vi "Scope_FPGA_Cavities_v00.vi"(0 "Scope IPs":T12, 9 "Scope":T8, 11 "Lock 4":T1, 12 "Cavities Data":u64[](array[numeric])) -> (3 "Scope OP Graph":cluster{dbl[], dbl[]}[](graph), 4 "Scope Cavities ON":bool, 8 "error":dbl[](array[numeric]), 10 "Scope Cavities":T13)   [LabVIEW 2010]
doc: "Creates an oscilliscope graph from the FIFO data, as well as packages data structures for FPGA_Cavities via the reference. (Needs tidying up). Based on a design by Ben Sparkes."
uses:
  Strict Type Defs/Control GUI v01.ctl
  Strict Type Defs/Slider and display.ctl
  Strict Type Defs/I16 white control.ctl
  Strict Type Defs/PII Gains.ctl
  Strict Type Defs/I2 gain slider.ctl
  Strict Type Defs/Thresh slider.ctl
  Strict Type Defs/Lock or Hold.ctl
  Strict Type Defs/Scan Freq Slider.ctl
  Strict Type Defs/DC polarity.ctl
  Strict Type Defs/Gains negative vertical.ctl
  Strict Type Defs/Lock Select 4.ctl
panel:
  in  "OPO A":T2={"Offset Error"=-0.004322033898305084, "Gain Error"=1, "Offset DC"=0.18926553672316412, "Gain DC"=1, "P Gain"=12, "P Bit Shift"=-7, "I Bit Shift"=-7, "I2 Bit Shift"=-27, "I Gain"=19, "I2 Gain"=0, "Lock Threshold"=66, "Lock"=FALSE, "Hold"=FALSE, "Scan Frequency"=19, "Scan Bit Shift"=-4, "DC negative"=FALSE, "Gains -ve "=FALSE} {"Scan Frequency" scale=1.0..30.0; "I2 Gain" scale=0.0..10.0; "I Gain" scale=0.0..50.0; "P Gain" scale=0.0..50.0; "Offset DC" scale=-5.0..0.5 scale format="%#_5f"; "Offset Error" scale=-0.01..0.005 scale format="%#_5f"}
  in  "OPO B":T2={"Offset Error"=-0.011977401129943503, "Gain Error"=4, "Offset DC"=1.29177966101695, "Gain DC"=1, "P Gain"=14, "P Bit Shift"=-8, "I Bit Shift"=-8, "I2 Bit Shift"=-27, "I Gain"=13, "I2 Gain"=0, "Lock Threshold"=67, "Lock"=FALSE, "Hold"=FALSE, "Scan Frequency"=10, "Scan Bit Shift"=-5, "DC negative"=TRUE, "Gains -ve "=FALSE} {"Scan Frequency" scale=1.0..30.0; "I2 Gain" scale=0.0..10.0; "I Gain" scale=0.0..50.0; "P Gain" scale=0.0..50.0; "Offset DC" scale=-5.1..3.0 scale format="%#_5f"; "Offset Error" scale format="%#_5f"}
  in  "MCC":T2={"Offset Error"=-0.006610169491525424, "Gain Error"=1, "Offset DC"=0.028813559322033905, "Gain DC"=1, "P Gain"=14, "P Bit Shift"=-8, "I Bit Shift"=-11, "I2 Bit Shift"=-27, "I Gain"=11, "I2 Gain"=0, "Lock Threshold"=20, "Lock"=FALSE, "Hold"=FALSE, "Scan Frequency"=10, "Scan Bit Shift"=-4, "DC negative"=TRUE, "Gains -ve "=TRUE} {"Scan Frequency" scale=1.0..30.0; "I2 Gain" scale=0.0..10.0; "I Gain" scale=0.0..50.0; "P Gain" scale=0.0..50.0; "Offset DC" scale=-0.1..0.2 scale format="%#_5f"; "Offset Error" scale=-0.02..0.01 scale format="%#_5f"}
  in  "Doubler":T2={"Offset Error"=-0.011581920903954804, "Gain Error"=1, "Offset DC"=-0.023163841807909608, "Gain DC"=1, "P Gain"=10, "P Bit Shift"=-7, "I Bit Shift"=-8, "I2 Bit Shift"=-27, "I Gain"=21, "I2 Gain"=0, "Lock Threshold"=12, "Lock"=FALSE, "Hold"=FALSE, "Scan Frequency"=8, "Scan Bit Shift"=-5, "DC negative"=FALSE, "Gains -ve "=FALSE} {"Scan Frequency" scale=1.0..30.0; "I2 Gain" scale=0.0..10.0; "I Gain" scale=0.0..50.0; "P Gain" scale=0.0..50.0; "Offset DC" scale=-0.1..0.1 scale format="%#_5f"; "Offset Error" scale=-0.05..0.05 scale format="%#_5f"}
  out "Scope OPs (for saving)":cluster{dbl[], i16[], i16[], i16[], i16[]}
  in  "Scope":T13={"Trigger Direction"=enum."minus-plus", "Delay"=0, "Aquisition Rate (Ticks)"=20, "Offset"=0, "Channel"=0, "Channel Selector"={"Channel 1"=0, "Channel 2"=0, "Channel 3"=0, "Channel 4"=0}}
  # "PII Gains"
  # "Lock"
  # "Error Signal"
  # "Monitor"
  # "Scan"
  # "DC positive"
  # "PII Gains"
  # "Lock"
  # "Error Signal"
  # "Monitor"
  # "Scan"
  # "DC positive"
  # "PII Gains"
  # "Lock"
  # "Error Signal"
  # "Monitor"
  # "Scan"
  # "DC positive"
  # "PII Gains"
  # "Lock"
  # "Error Signal"
  # "Monitor"
  # "Scan"
  # "DC positive"
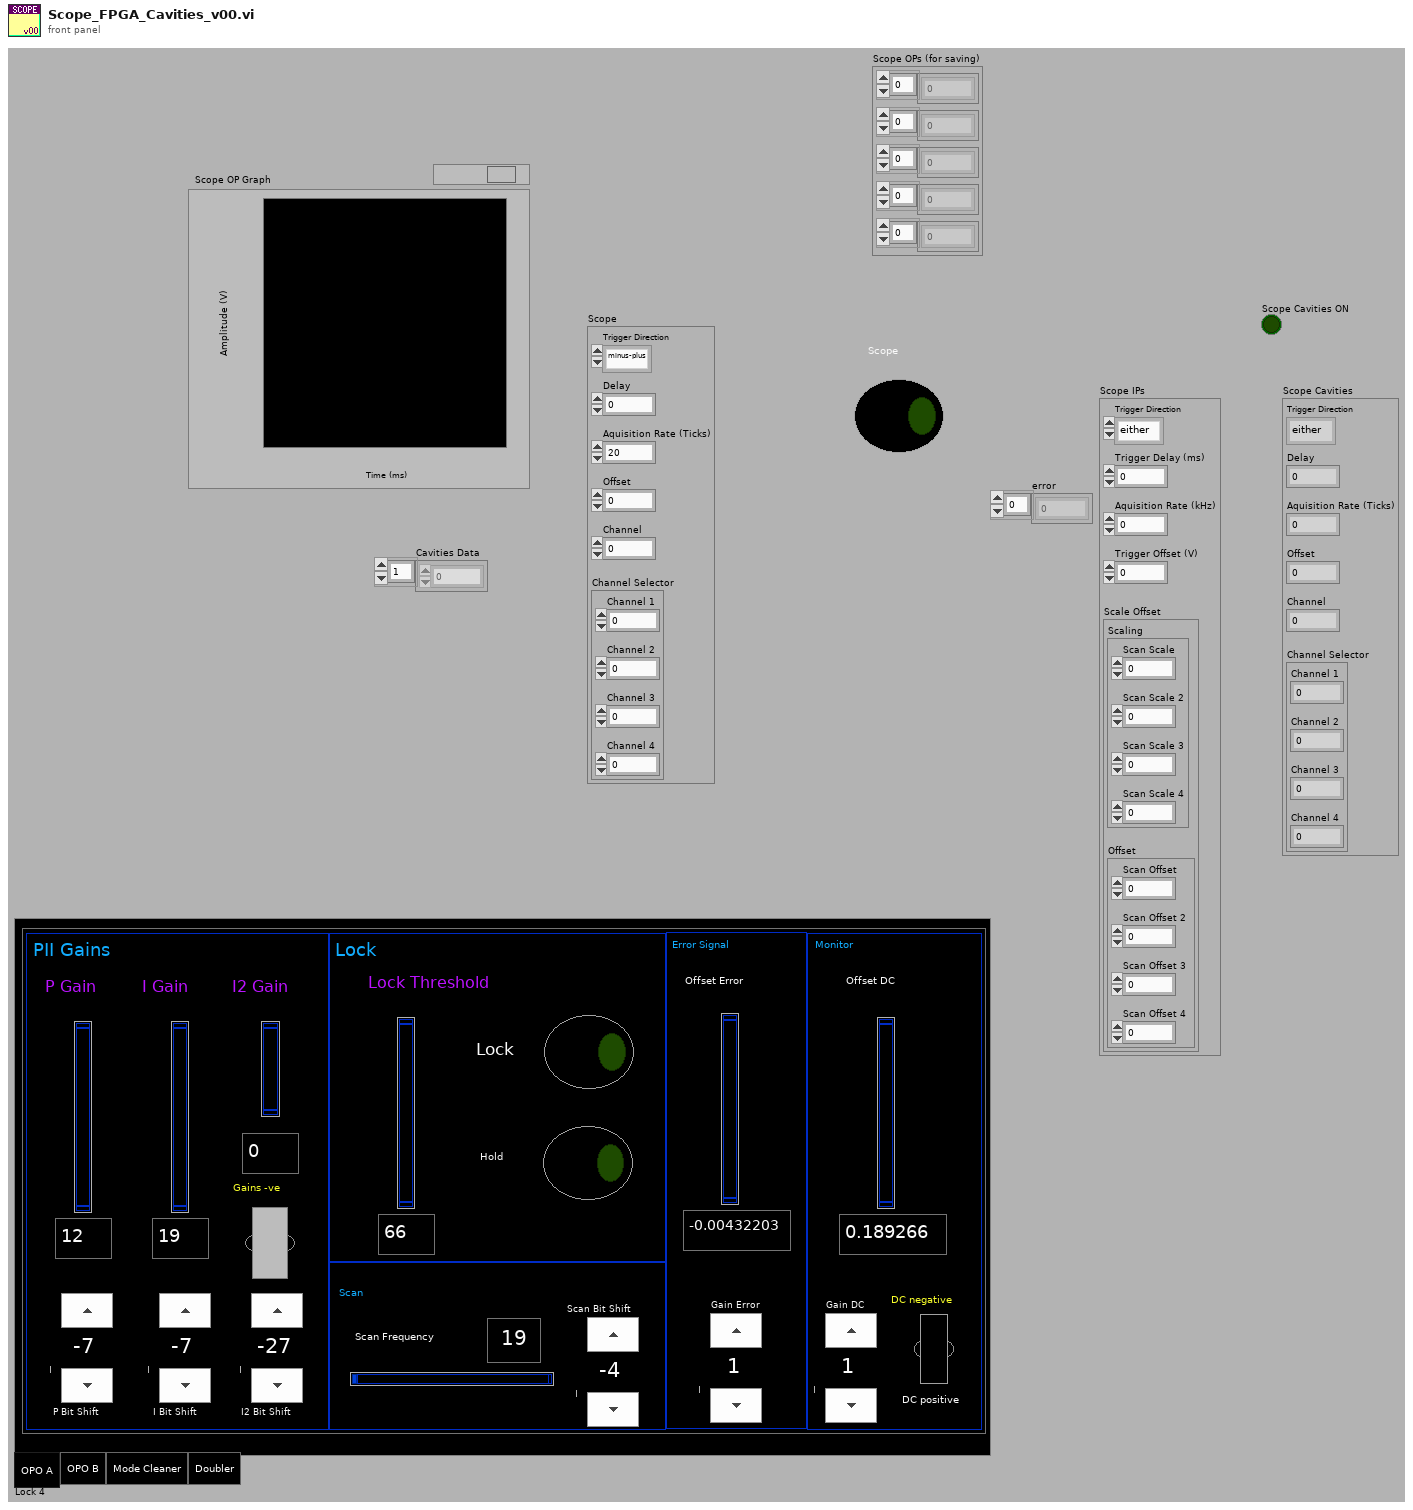
[diagram p1: front panel]
types:
  T1 = typedef "Lock Select 4.ctl" = enum32{"OPO A", "OPO B", "Mode Cleaner", "Doubler"}
  T2 = typedef "Control GUI v01.ctl" = cluster{"Offset Error":T3, "Gain Error":T4, "Offset DC":T3, "Gain DC":T4, "P Gain":T5, "P Bit Shift":T4, "I Bit Shift":T4, "I2 Bit Shift":T4, "I Gain":T5, "I2 Gain":T6, "Lock Threshold":T7, "Lock":T8, "Hold":T8, "Scan Frequency":T9, "Scan Bit Shift":T4, "DC negative":T10, "Gains -ve ":T11}
  T3 = typedef "Slider and display.ctl" = dbl
  T4 = typedef "I16 white control.ctl" = i16
  T5 = typedef "PII Gains.ctl" = i32
  T6 = typedef "I2 gain slider.ctl" = i32
  T7 = typedef "Thresh slider.ctl" = i16
  T8 = typedef "Lock or Hold.ctl" = bool
  T9 = typedef "Scan Freq Slider.ctl" = u16
  T10 = typedef "DC polarity.ctl" = bool
  T11 = typedef "Gains negative vertical.ctl" = bool
  T12 = cluster{"Trigger Direction":enum8{"either", "minus-plus", "plus-minus"}, "Trigger Delay (ms)":dbl, "Aquisition Rate (kHz)":dbl, "Trigger Offset (V)":dbl, "Scale Offset":cluster{"Scaling":cluster{"Scan Scale":i16, "Scan Scale 2":i16, "Scan Scale 3":i16, "Scan Scale 4":i16}, "Offset":cluster{"Scan Offset":i16, "Scan Offset 2":i16, "Scan Offset 3":i16, "Scan Offset 4":i16}}}
  T13 = cluster{"Trigger Direction":enum8{"either", "minus-plus", "plus-minus"}, "Delay":u32, "Aquisition Rate (Ticks)":u32, "Offset":i16, "Channel":i32, "Channel Selector":cluster{"Channel 1":i32, "Channel 2":i32, "Channel 3":i32, "Channel 4":i32}}
  T14 = cluster{"Channel 1":i32, "Channel 2":i32, "Channel 3":i32, "Channel 4":i32}
  T15 = cluster{"Scan Scale":i16, "Scan Scale 2":i16, "Scan Scale 3":i16, "Scan Scale 4":i16}
  T16 = cluster{"Scan Offset":i16, "Scan Offset 2":i16, "Scan Offset 3":i16, "Scan Offset 4":i16}
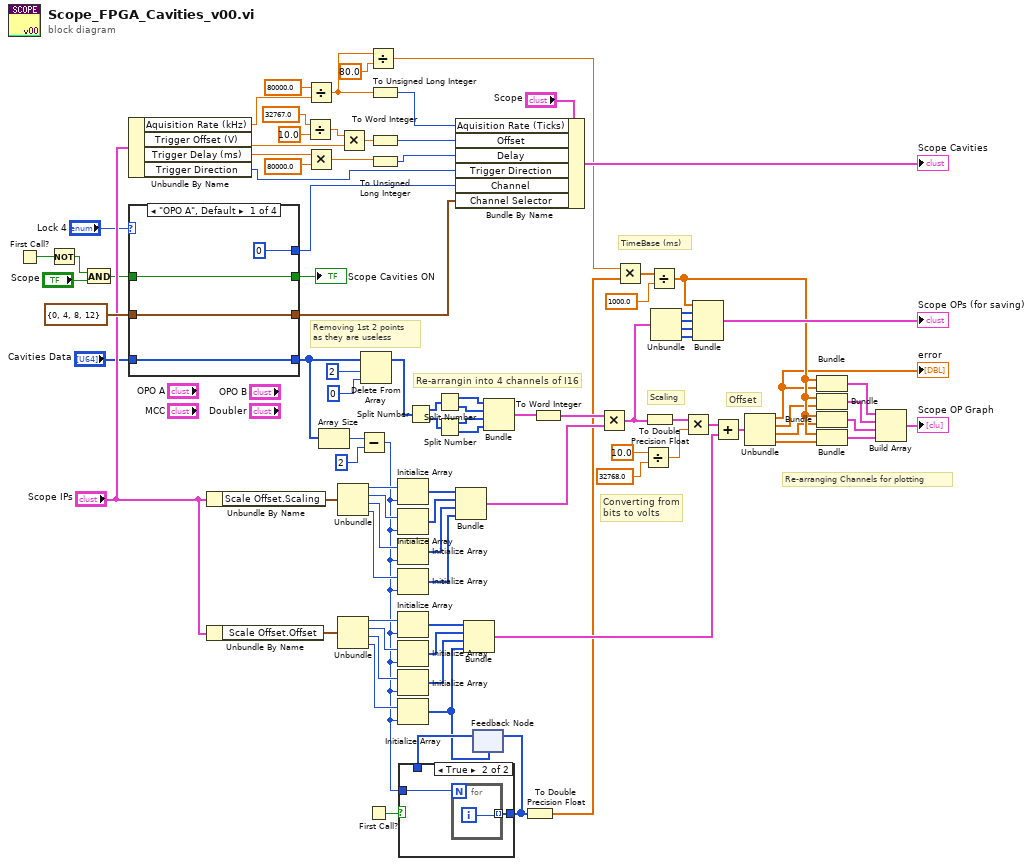
[diagram p0: block diagram]
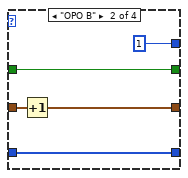
[diagram p3: hidden frame]
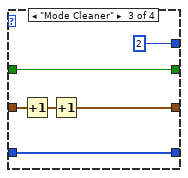
[diagram p4: hidden frame]
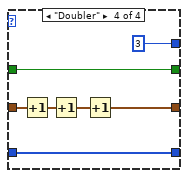
[diagram p5: hidden frame]
diagram:
  # "TimeBase (ms)"
  # "Re-arranging Channels for plotting"
  # "Re-arrangin into 4 channels of I16"
  # "Converting from\nbits to volts"
  # "Offset"
  # "Scaling"
  # "Removing 1st 2 points\nas they are useless"
  n1 = First Call?() -> (First Call?: T/F=w9:bool)
  n2 = Not(x=w9) -> (.not. x?=w4:bool)
  n3 = And(x=w4, y="Scope") -> (x .and. y?=w7:T8)
  n4 = Unbundle By Name("Scope IPs") -> ("Aquisition Rate (kHz)"=w92:dbl, "Trigger Offset (V)"=w87:dbl, "Trigger Delay (ms)"=w85:dbl, "Trigger Direction"=w10:enum8{"either", "minus-plus", "plus-minus"})
  n5 = case shown="\"OPO A\", Default" "Lock 4" {
    tunnel: T14 {"Channel 1"=0, "Channel 2"=4, "Channel 3"=8, "Channel 4"=12} ("Channel Selector") -> [w97 w100 w106 w113]
    tunnel: [w97 w99 w104 w110] -> w83
    tunnel: [0 1 2 3] -> w82
    tunnel: [w96 w102 w108 w115] -> w16
    tunnel: "Cavities Data" -> [w96 w102 w108 w115]
    tunnel: [w94 w98 w103 w109] -> w8
    tunnel: w7 -> [w94 w98 w103 w109]
    frame "OPO A", Default {
    }
    frame "OPO B" {
      n6 = Increment(x=w100) -> (x+1=w99:T14)
    }
    frame "Mode Cleaner" {
      n7 = Increment(x=w106) -> (x+1=w105:T14)
      n8 = Increment(x=w105) -> (x+1=w104:T14)
    }
    frame "Doubler" {
      n9 = Increment(x=w113) -> (x+1=w112:T14)
      n10 = Increment(x=w112) -> (x+1=w111:T14)
      n11 = Increment(x=w111) -> (x+1=w110:T14)
    }
  }
  "Scope Cavities ON" <- w8
  n12 = Unbundle By Name("Scope IPs") -> ("Scale Offset.Scaling"=w47:T15)
  n13 = Unbundle By Name("Scope IPs") -> ("Scale Offset.Offset"=w31:T16)
  n14 = Divide(x=32767.0, y=10.0) -> (x/y=w90:dbl)
  n15 = Divide(x=80000.0, y=w92) -> (x/y=w80:dbl)
  n16 = Multiply(x=w85, y=80000.0) -> (x*y=w86:dbl)
  n17 = Array Size(array=w16) -> (size(s)=w76:i32)
  n18 = Unbundle(w47) -> ("Scan Scale"=w44:i16, "Scan Scale 2"=w43:i16, "Scan Scale 3"=w45:i16, "Scan Scale 4"=w46:i16)
  n19 = Unbundle(w31) -> ("Scan Offset"=w30:i16, "Scan Offset 2"=w34:i16, "Scan Offset 3"=w33:i16, "Scan Offset 4"=w32:i16)
  n20 = Multiply(x=w90, y=w87) -> (x*y=w91:dbl)
  n21 = Subtract(x=w76, y=2) -> (x-y=w1:i32)
  n22 = Delete From Array(array=w16, length=2, index=0) -> (array with subset deleted=w22:u64[])  [unwired: 1 out]
  n23 = First Call?() -> (First Call?: T/F=w50:bool)
  n24 = Divide(x=w80, y=80.0) -> (x/y=w3:dbl)
  n25 = To Unsigned Long Integer(number=w80) -> (unsigned 32bit integer=w13:u32)
  n26 = To Word Integer(number=w91) -> (16bit integer=w12:i16)
  n27 = To Unsigned Long Integer(number=w86) -> (unsigned 32bit integer=w11:u32)
  n28 = Initialize Array(w44, w1) -> (w42:i16[])
  n29 = Initialize Array(w43, w1) -> (w41:i16[])
  n30 = Initialize Array(w45, w1) -> (w40:i16[])
  n31 = Initialize Array(w46, w1) -> (w39:i16[])
  n32 = Initialize Array(w30, w1) -> (w35:i16[])
  n33 = Initialize Array(w34, w1) -> (w36:i16[])
  n34 = Initialize Array(w33, w1) -> (w37:i16[])
  n35 = Initialize Array(w32, w1) -> (w51:i16[])
  n36 = Split Number(x=w22) -> (hi(x)=w24:u32[], lo(x)=w23:u32[])
  n37 = Split Number(x=w24) -> (hi(x)=w72:u16[], lo(x)=w73:u16[])
  n38 = Split Number(x=w23) -> (hi(x)=w74:u16[], lo(x)=w75:u16[])
  n39 = Bundle By Name(cluster="Scope", "Aquisition Rate (Ticks)"=w13, "Offset"=w12, "Delay"=w11, "Trigger Direction"=w10, "Channel"=w82, "Channel Selector"=w83) -> (→"Scope Cavities":T13)
  n40 = Bundle(w42, w41, w40, w39) -> (w38:cluster{i16[], i16[], i16[], i16[]})  [unwired: 1 out]
  n41 = Bundle(w35, w36, w37, w51) -> (w29:cluster{i16[], i16[], i16[], i16[]})  [unwired: 1 out]
  n42 = feedback #1(w51) -> (w52:i32[])
  n43 = case shown="True" w50 {
    tunnel: w1 -> [_ w118]
    tunnel: [w116 w117] -> w53
    tunnel: w52 -> [w116 _]
    frame False {
    }
    frame True {
      n44 = for {
        N: w118 -> [_]
        tunnel: [w119] -> w117 mode=indexing
        i -> [w119]
      }
    }
  }
  n45 = feedback-in #1(w53) -> ()
  n46 = Bundle(w72, w73, w74, w75) -> (w48:cluster{u16[], u16[], u16[], u16[]})  [unwired: 1 out]
  n47 = To Double Precision Float(number=w53) -> (double precision float=w2:dbl[])
  n48 = To Word Integer(number=w48) -> (16bit integer=w49:cluster{i16[], i16[], i16[], i16[]})
  n49 = Multiply(x=w49, y=w38) -> (x*y=w65:cluster{i16[], i16[], i16[], i16[]})
  n50 = Multiply(x=w3, y=w2) -> (x*y=w54:dbl[])
  n51 = Divide(x=10.0, y=32768.0) -> (x/y=w17:dbl)
  n52 = To Double Precision Float(number=w65) -> (double precision float=w18:cluster{dbl[], dbl[], dbl[], dbl[]})
  n53 = Divide(x=w54, y=1000.0) -> (x/y=w70:dbl[])
  n54 = Unbundle(w65) -> (w66:i16[], w67:i16[], w68:i16[], w69:i16[])
  n55 = Multiply(x=w18, y=w17) -> (x*y=w27:cluster{dbl[], dbl[], dbl[], dbl[]})
  n56 = Bundle(w70, w66, w67, w68, w69) -> (→"Scope OPs (for saving)":cluster{dbl[], i16[], i16[], i16[], i16[]})  [unwired: 1 in]
  n57 = Add(x=w27, y=w29) -> (x+y=w28:cluster{dbl[], dbl[], dbl[], dbl[]})
  n58 = Unbundle(w28) -> (w56:dbl[], w57:dbl[], w58:dbl[], w59:dbl[])
  "error" <- w56
  n59 = Bundle(w70, w56) -> (w60:cluster{dbl[], dbl[]})  [unwired: 1 in]
  n60 = Bundle(w70, w57) -> (w61:cluster{dbl[], dbl[]})  [unwired: 1 in]
  n61 = Bundle(w70, w58) -> (w62:cluster{dbl[], dbl[]})  [unwired: 1 in]
  n62 = Bundle(w70, w59) -> (w63:cluster{dbl[], dbl[]})  [unwired: 1 in]
  n63 = Build Array(w60, w61, w62, w63) -> (→"Scope OP Graph":cluster{dbl[], dbl[]}[])
